vi "Write Active.vi"(10 "Active?":bool, 11 "Log Sinks in":refnum<class "Log Sinks.lvclass">) -> (3 "Log Sinks out":refnum<class "Log Sinks.lvclass">)   [LabVIEW 2019, in "TSC Event Logger.lvlib" / "Log Sinks.lvclass"]
doc: "Write if the sink is currently active.\n\n<b>Code Developed By:</b>\nTechnology Service Corporation\nBloomington, IN 47403\nwww.tsc.com/atcs\n\nDeveloper:\nDaniel Coons"
uses:
  Log Sinks.lvclass
  Log Sinks.lvclass/Log Sinks.ctl
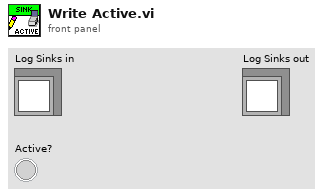
[diagram p1: front panel]
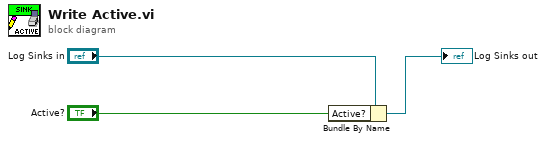
[diagram p0: block diagram]
diagram:
  n1 = Bundle By Name(cluster="Log Sinks in", "Active?"="Active?") -> (→"Log Sinks out":refnum<class "Log Sinks.lvclass">)
